vi "声发射信号处理.vi"(0 "输入信号":dbl[](array[numeric])=[0.0, 1.0, 0.0, 4.0, 0.0, 4.0, 0.0, 1.0, 0.0, 3.0, 0.0, 4.0, 0.0, 1.0, 0.0, 2.0, 3.0] caption="X", 5 "阈值":dbl format="%0.2f", 9 "下一个事件":bool) -> (1 "自功率谱":dbl[](graph), 2 "XY图":cluster{"Locations":dbl[], "振幅":dbl[]}[](graph), 4 "RMS value":dbl caption="RMS" format="%0.5f", 6 "幅值":dbl, 8 "Locations":dbl[](array[numeric]) caption="位置", 10 "事件个数":i32, 12 "自相关":dbl[](graph), 13 "事件":T1(array[cluster]), 14 "表格控件":string[][](table), 15 "振幅":dbl[](array[numeric]))   [LabVIEW 2014]
uses:
  <vilib>/Analysis/2dsp.llb/1D Auto Correlation (DBL).vi
  <vilib>/Analysis/NI_AAL_SigProc.lvlib
  <vilib>/Analysis/NI_AALPro.lvlib
panel:
  in  "数组":string[](array[string])
  in  "事件计数":i32=-1
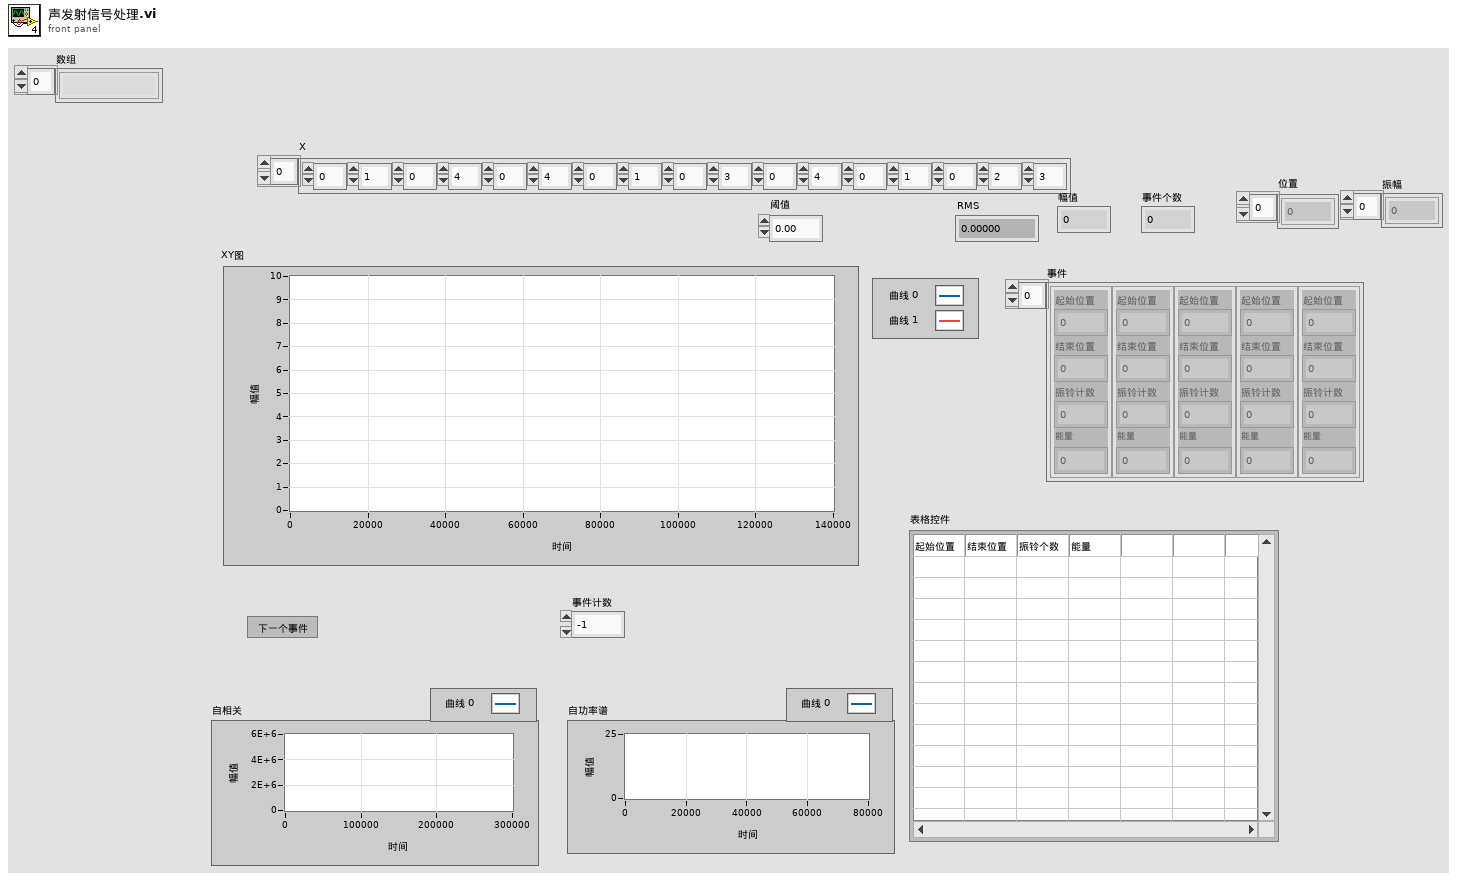
[diagram p1: front panel]
types:
  T1 = cluster{"起始位置":i32, "结束位置":i32, "振铃计数":i32, "能量":i32}[]
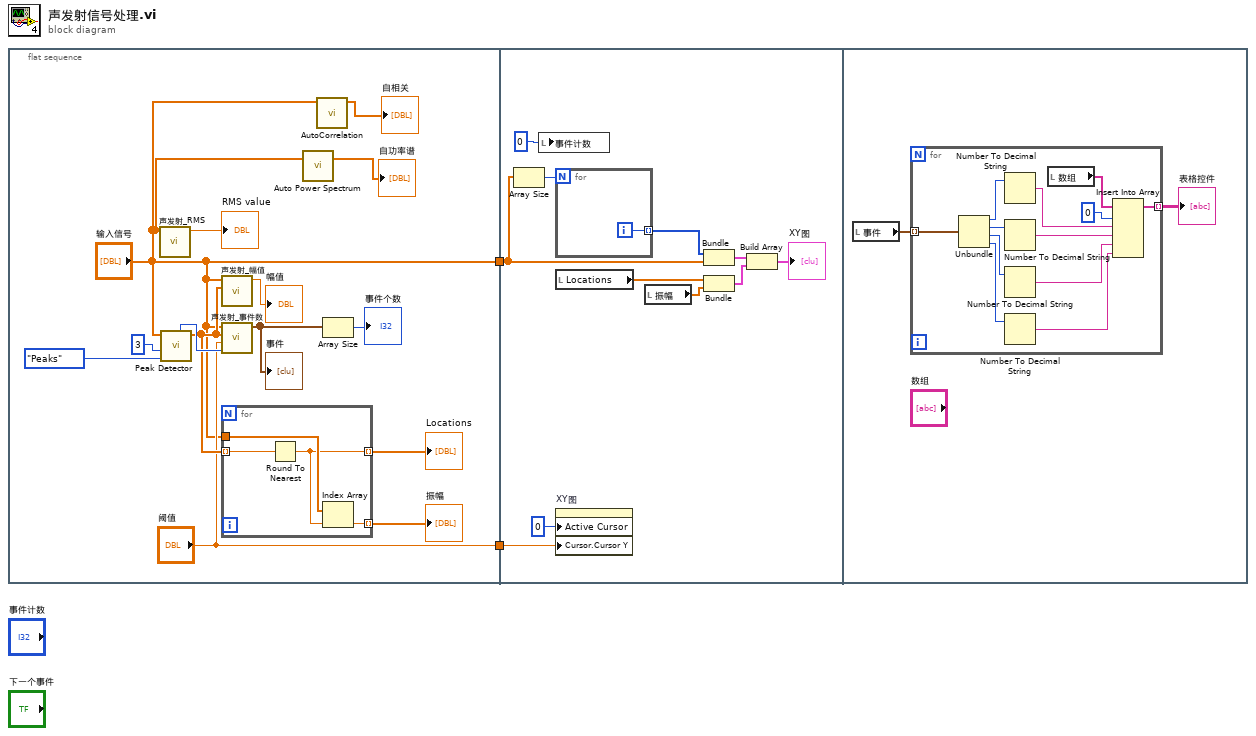
[diagram p0: block diagram]
diagram:
  n1 = flat-sequence {
    tunnel: ["输入信号"] -> w2
    tunnel: ["阈值"] -> w1
    tunnel: w2 -> [w29]
    tunnel: w1 -> [w21]
    frame #0 {
      n2 = call "声发射_RMS.vi"("输入信号"="输入信号") -> ("RMS value"=→"RMS value":dbl)  [unwired: 10 in]
      n3 = call <vilib>:"Peak Detector.vi"("peaks/valleys"=enum32{"Peaks", "Valleys"}."Peaks", "width"=3, "X"="输入信号") -> ("Locations"=w9:dbl[], "# found"=w16:i32)  [unwired: 4 in, 3 out]
      n4 = call "声发射_幅值.vi"("波峰位置"=w9, "数据"="输入信号") -> ("幅值"=→"幅值":dbl)  [unwired: 9 in]
      n5 = call "声发射_事件数.vi"("波峰个数"=w16, "阈值"="阈值", "位置"=w9, "数据"="输入信号") -> ("事件数组"=w13:T1)  [unwired: 7 in]
      "事件" <- w13
      n6 = for {
        tunnel: w9 -> [w20] mode=indexing
        tunnel: [w18] -> w8 mode=indexing
        tunnel: "输入信号" -> [w19]
        tunnel: [w17] -> w7 mode=indexing
        n7 = Round To Nearest(number=w20) -> (nearest integer value=w18:dbl)
        n8 = Index Array(array=w19, index=w18) -> (element=w17:dbl)
      }
      "Locations" <- w8
      "振幅" <- w7
      n9 = call <vilib>:"Auto Power Spectrum.vi"("Signal (V)"="输入信号") -> ("Power Spectrum (V^2 rms)"=→"自功率谱":dbl[])  [unwired: 1 in, 1 out]
      n10 = call-poly <vilib>:"AutoCorrelation.vi"("X"="输入信号") -> ("Rxx"=→"自相关":dbl[])  [unwired: 9 in, 1 out]
      n11 = Array Size(array=w13) -> (size(s)=→"事件个数":i32)
    }
    frame #1 {
      n12 = Array Size(array=w29) -> (size(s)=w31:i32)
      n13 = local write "事件计数"(0 ("事件计数")) -> ()
      n14 = for {
        N: w31 -> [_]
        tunnel: [w32] -> w30 mode=indexing
        i -> [w32]
      }
      n15 = local read "Locations"() -> (w25:dbl[])
      n16 = property on="XY图" class="XYGraph (严格)"("Active Cursor"=u32 0 ("活动游标"), "Cursor.Cursor Y"=w21) -> ()  [unwired: 2 in, 2 out]
      n17 = local read "振幅"() -> (w24:dbl[])
      n18 = Bundle(w30, "输入信号"=w29) -> (w28:cluster{i32[], "输入信号":dbl[]})  [unwired: 1 in]
      n19 = Bundle("Locations"=w25, "振幅"=w24) -> (w27:cluster{"Locations":dbl[], "振幅":dbl[]})  [unwired: 1 in]
      n20 = Build Array(w28, w27) -> (→"XY图":cluster{"Locations":dbl[], "振幅":dbl[]}[])
    }
    frame #2 {
      n21 = local read "事件"() -> (w34:T1)
      n22 = for {
        tunnel: w34 -> [w46] mode=indexing
        tunnel: [w35] -> w33 mode=indexing
        n23 = Unbundle(w46) -> ("起始位置"=w44:i32, "结束位置"=w42:i32, "振铃计数"=w41:i32, "能量"=w40:i32)
        n24 = Number To Decimal String(number=w44) -> (decimal integer string=w43:string)  [unwired: 1 in]
        n25 = Number To Decimal String(number=w42) -> (decimal integer string=w39:string)  [unwired: 1 in]
        n26 = Number To Decimal String(number=w41) -> (decimal integer string=w38:string)  [unwired: 1 in]
        n27 = Number To Decimal String(number=w40) -> (decimal integer string=w37:string)  [unwired: 1 in]
        n28 = local read "数组"() -> (w36:string[])
        n29 = Insert Into Array(array=w36, index=0 ("索引"), new element #1=w43, new element #2=w39, new element #3=w38, new element #4=w37) -> (w35:string[])
      }
      "表格控件" <- w33
    }
  }
